vi "Process.vi"(8 "error in (no error)":errorcluster, 10 "Pound in":refnum<class "Pound.lvclass">, 11 "Qbus in":refnum<class "Qbus.lvclass">) -> (0 "error out":errorcluster)   [LabVIEW 2017, in "Controller.lvlib"]
doc: "This process performs device-wide operations, such as restarting all processes during a reboot and monitoring that each process starts up successfully."
uses:
  <vilib>/addons/InsightCM/Devices/Shared/Common/Controller/Controller.lvlib
  <vilib>/addons/Qbus/Qbus.lvclass
  <vilib>/NI/Software Watchdog/Pound/Pound.lvclass
  <vilib>/addons/InsightCM/Devices/Shared/Common/Controller/controls/config.ctl
  <vilib>/addons/BlinkProcess/controls/mode.ctl
  <vilib>/addons/InsightCM/MessageBus/MessageLibrary/Device/controls/DeviceInvalidConfigurationBroadcastBody.ctl
  <vilib>/addons/InsightCM/Devices/Shared/Common/ServerComm/controls/ConnectionStatus.ctl
  <vilib>/addons/InsightCM/Devices/Shared/Cms/CmsAcquisition/controls/StopAcquisitionRequest.ctl
  <vilib>/addons/InsightCM/Devices/Shared/Common/Controller/controls/operations.ctl
  <vilib>/addons/TraceLogger/TraceLogger.lvlib
  <vilib>/NI/Software Watchdog/Watchdog/Watchdog.lvclass
  <vilib>/addons/InsightCM/Devices/Shared/Common/ServerComm/ServerComm.lvlib
  <vilib>/addons/BlinkProcess/BlinkProcess.lvlib
  <vilib>/addons/InsightCM/Utilities/GlobalConfiguration/GlobalConfiguration.lvlib
  <vilib>/addons/InsightCM/Devices/Shared/Cms/CmsAcquisition/CmsAcquisition.lvlib
  <vilib>/addons/InsightCM/Devices/Shared/Cms/CmsBurstMode/BurstMode.lvlib
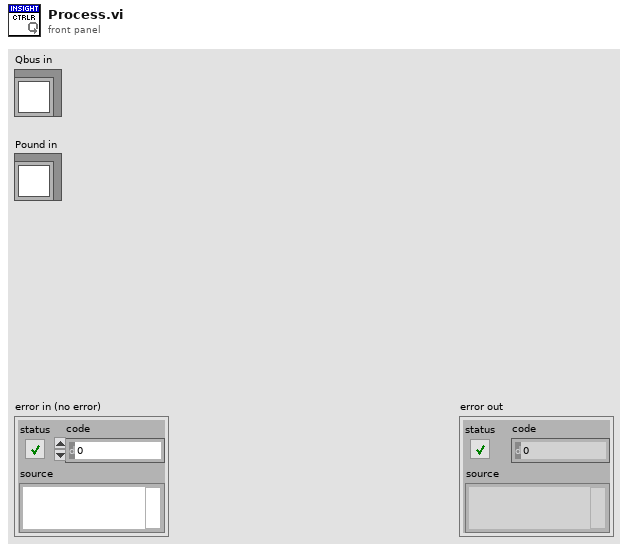
[diagram p1: front panel]
types:
  T1 = typedef "Controller.lvlib/config.ctl" = cluster{"Online":bool, "SafeMode":bool, "InvalidConfig":string, "ShutdownReason":string, "ScheduledShutdown":bool}
  T2 = typedef "BlinkProcess.lvlib/mode.ctl" = enum16{"Normal", "Error", "On", "Off", "Custom"}
  T3 = typedef "DeviceInvalidConfigurationBroadcastBody.ctl" = cluster{"DeviceName":string, "Description":string}
  T4 = typedef "ServerComm.lvlib/ConnectionStatus.ctl" = enum16{"Offline", "NotAuthorized", "Online"}
  T5 = typedef "CmsAcquisition.lvlib/StopAcquisitionRequest.ctl" = cluster{"Reason":string, "State":variant}
  T6 = typedef "Controller.lvlib/operations.ctl" = enum16{"Unknown", "Startup", "Expected Shutdown"}
  T7 = typedef "R2_Device.ctl" = cluster{"Id":string, "Name":string, "DeviceType":string, "HardwareName":string, "IpAddress":string, "HardwareInfo":T8[], "ApplicationType":string, "ApplicationVersion":string, "EquipmentIds":string[], "ConfigurationVersion":string, "State":T9, "Properties":T8[], "DataGroups":T10[], "BurstModeTrigger":T14}
  T8 = typedef "KeyValuePair.ctl" = cluster{"Key":string, "Value":string}
  T9 = typedef "DeviceState.ctl" = cluster{"Disabled":bool}
  T10 = typedef "R2_DataGroup.ctl" = cluster{"Name":string, "OperatingStates":T11[], "Properties":T8[], "EquipmentIds":string[], "AssetNodeId":string}
  T11 = typedef "OperatingState.ctl" = cluster{"Name":string, "Properties":T8[], "Triggers":T12[]}
  T12 = typedef "Trigger.ctl" = cluster{"Type":string, "Expression":string, "Conditions":T13[]}
  T13 = typedef "Condition.ctl" = cluster{"Source":string, "Type":string, "Operator":string, "CompareTo":string, "DwellSeconds":dbl}
  T14 = typedef "BurstModeTrigger.ctl" = cluster{"Trigger":T12, "SampleRate":string, "AcquisitionLength":string}
  T15 = typedef "Message.ctl" = cluster{"Header":T16, "Body":u8[]}
  T16 = typedef "MessageHeader.ctl" = cluster{"MessageName":string, "Timestamp":i64, "CorrelationId":string, "ContentType":string, "RoutingKey":string, "Properties":T8[]}
  T17 = typedef "BurstMode.lvlib/InitiateBurstMode.ctl" = cluster{"Group":string, "Acq Reason":string}
  T18 = typedef "CmsAcquisition.lvlib/StopAcquisitionResponse.ctl" = cluster{"Reason":string, "Acquisition Stopped":bool, "State":variant}
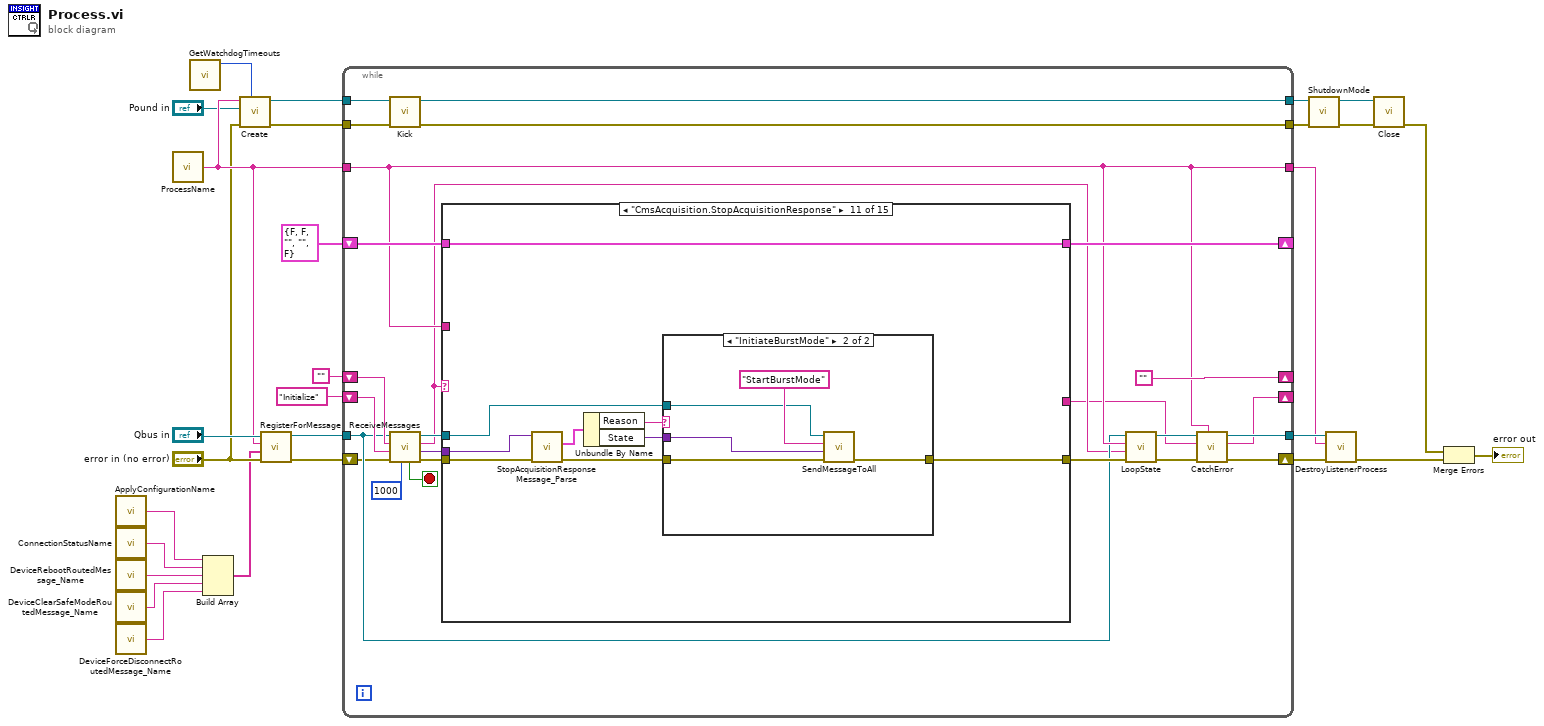
[diagram p0: block diagram]
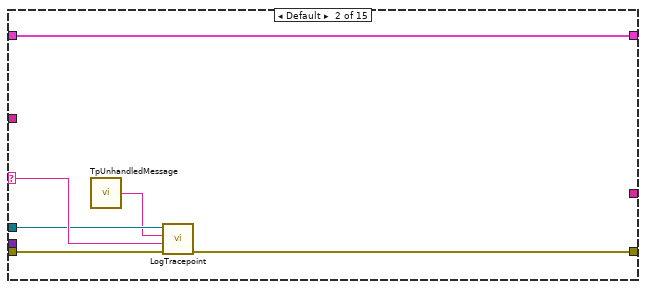
[diagram p3: hidden frame]
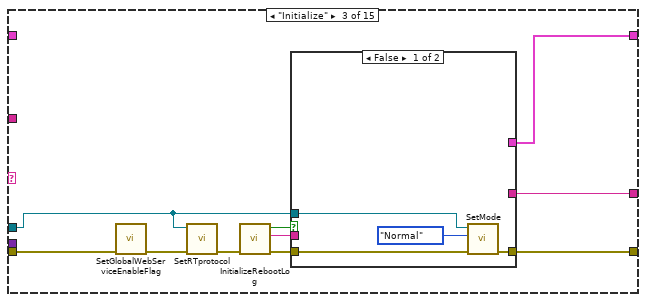
[diagram p4: hidden frame]
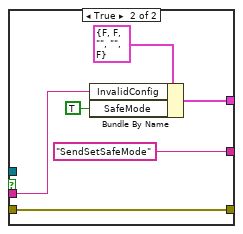
[diagram p5: hidden frame]
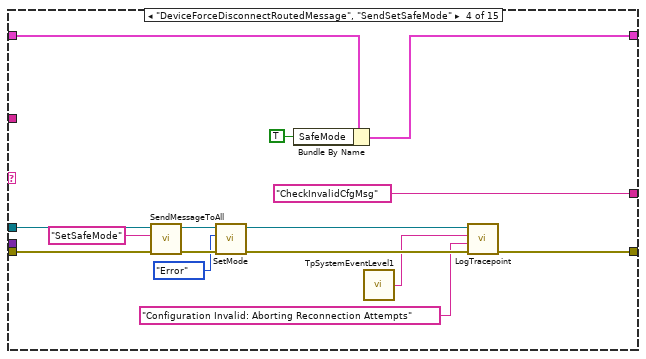
[diagram p6: hidden frame]
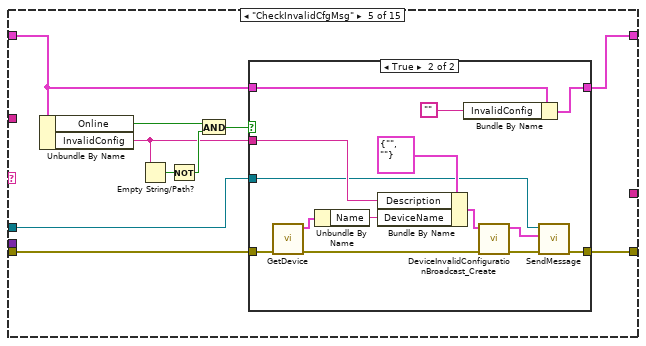
[diagram p7: hidden frame]
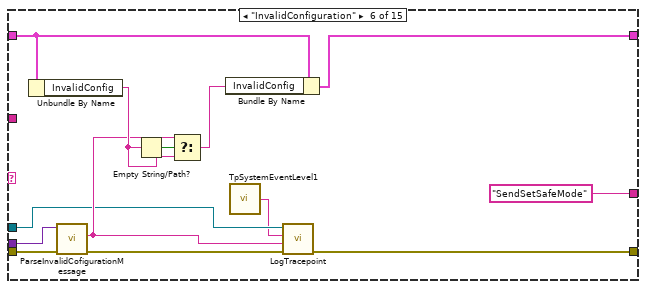
[diagram p9: hidden frame]
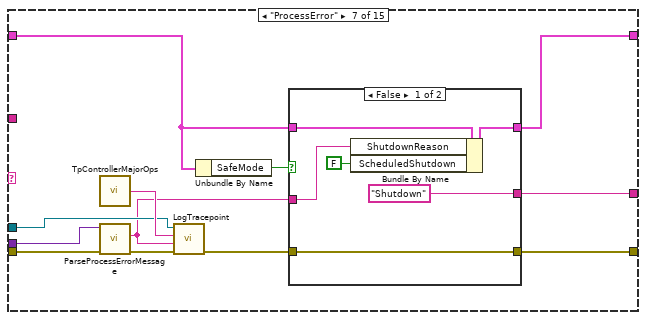
[diagram p10: hidden frame]
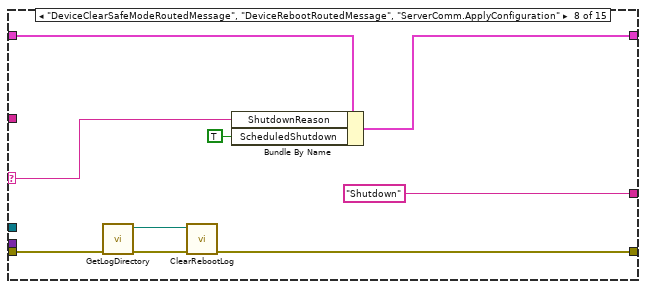
[diagram p12: hidden frame]
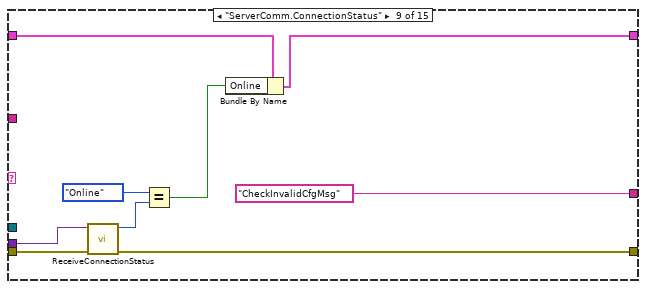
[diagram p13: hidden frame]
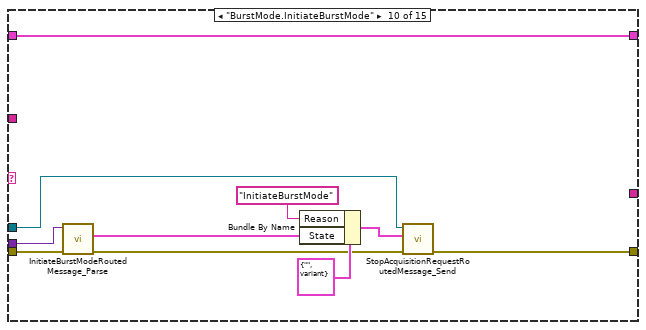
[diagram p14: hidden frame]
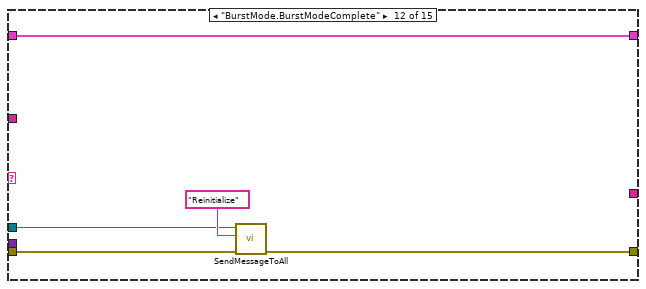
[diagram p16: hidden frame]
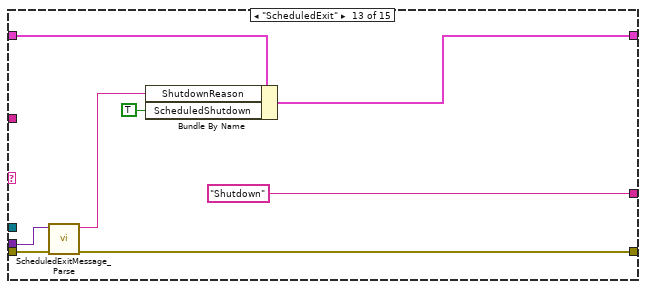
[diagram p17: hidden frame]
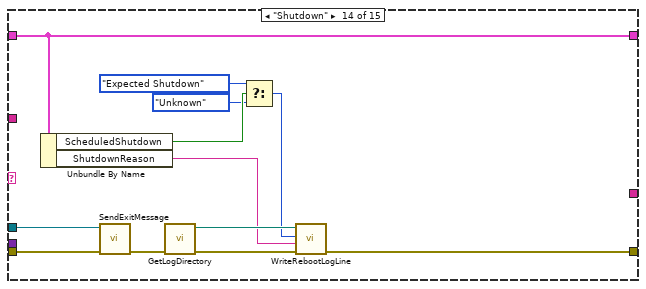
[diagram p18: hidden frame]
diagram:
  n1 = call <vilib>:"ApplyConfigurationName.vi"() -> ("message name"=w6:string)  [unwired: 5 in]
  n2 = call <vilib>:"ConnectionStatusName.vi"() -> ("message name"=w5:string)  [unwired: 5 in]
  n3 = call <vilib>:"DeviceRebootRoutedMessage_Name.vi"() -> ("MessageName"=w4:string)  [unwired: 5 in]
  n4 = call <vilib>:"DeviceClearSafeModeRoutedMessage_Name.vi"() -> ("MessageName"=w3:string)  [unwired: 5 in]
  n5 = call <vilib>:"DeviceForceDisconnectRoutedMessage_Name.vi"() -> ("MessageName"=w2:string)  [unwired: 5 in]
  n6 = call <vilib>:"ProcessName.vi"() -> ("ProcessName"=w19:string)  [unwired: 5 in]
  n7 = call <vilib>:"GetWatchdogTimeouts.vi"() -> ("software timeout"=w1:u32)  [unwired: 10 in, 1 out]
  n8 = Build Array(w6, w5, w4, w3, w2) -> (w7:string[])
  n9 = call <vilib>:"Create.vi"("Execution Timeout (ms)"=w1, "error in (no error)"="error in (no error)", "Pound"="Pound in", "Name"=w19) -> ("error out"=w13:errorcluster, "Watchdog"=w18:refnum<data-value>)  [unwired: 6 in]
  n10 = call <vilib>:"RegisterForMessage.vi"("error in (no error)"="error in (no error)", "message names"=w7, "process name"=w19, "Qbus in"="Qbus in") -> ("error in (no error)"=w27:errorcluster, "Qbus out"=w26:refnum<class "Qbus.lvclass">)  [unwired: 6 in]
  n11 = while {
    shift-right: [""] -> _
    shift-left: "" -> [w52]
    tunnel: w26 -> [w39]
    tunnel: w19 -> [w40]
    tunnel: [w43] -> w24
    tunnel: [w40] -> w23
    shift-right: [w42] -> _
    shift-left: "Initialize" -> [w47]
    shift-right: [w45] -> _
    shift-left: T1 {"Online"=FALSE, "SafeMode"=FALSE, "InvalidConfig"="", "ShutdownReason"="", "ScheduledShutdown"=FALSE} ("config") -> [w46]
    tunnel: w18 -> [w38]
    tunnel: [w37] -> w15
    tunnel: w13 -> [w36]
    tunnel: [w34] -> w12
    shift-right: [w44] -> w25
    shift-left: w27 -> [w35]
    stop <- w53 stop-if-true
    n12 = call <vilib>:"Kick.vi"("error in (no error)"=w36, "Watchdog"=w38) -> ("error out"=w34:errorcluster, "Watchdog"=w37:refnum<data-value>)  [unwired: 8 in]
    n13 = call <vilib>:"ReceiveMessages.vi"("Timeout(100)"=1000, "error in (no error)"=w35, "Priority Action"=w47, "Default Action"=w52, "Qbus in"=w39) -> ("error out"=w51:errorcluster, "MsgValue"=w48:variant, "Action"=w31:string, "Qbus out"=w49:refnum<class "Qbus.lvclass">, "Exit"=w53:bool)  [unwired: 2 in]
    n14 = case shown="\"CmsAcquisition.StopAcquisitionResponse\"" w31 {
      selector: w31 -> [_ w58 _ _ _ _ _ w156 _ _ _ _ _ _ _]
      tunnel: w51 -> [w54 w60 w65 w92 w106 w135 w144 w159 w173 w176 w188 w200 w211 w221 w224]
      tunnel: w49 -> [_ w57 w66 w91 w99 w124 w141 _ _ w182 w190 w201 _ w219 _]
      tunnel: [w54 w59 w69 w85 w105 w126 w146 w157 w169 w178 w191 w199 w204 w220 w224] -> w41
      tunnel: w48 -> [_ _ _ _ _ w134 w143 _ w172 w177 w189 _ w210 _ _]
      tunnel: w46 -> [w55 w61 _ w89 w98 w133 w137 w163 w171 w183 w192 w203 w208 w217 w225]
      tunnel: [w55 w61 w70 w88 w97 w130 w136 w162 w170 w183 w192 w203 w207 w217 w225] -> w45
      tunnel: w40 -> [_ _ _ _ _ _ _ _ _ _ _ _ _ _ _]
      tunnel: [_ _ w62 "CheckInvalidCfgMsg" ("error string") _ "SendSetSafeMode" ("log string") w138 "Shutdown" ("error string") "CheckInvalidCfgMsg" ("error string") _ _ _ "Shutdown" ("error string") _ _] -> w29
      frame "" {
      }
      frame Default {
        n15 = call <vilib>:"TpUnhandledMessage.vi"() -> ("tracepoint name"=w56:string)  [unwired: 5 in]
        n16 = call <vilib>:"LogTracepoint.vi"("error in (no error)"=w60, "log string"=w58, "tracepoint"=w56, "qbus in"=w57) -> ("error out"=w59:errorcluster)  [unwired: 6 in, 1 out]
      }
      frame "Initialize" {
        n17 = call <vilib>:"SetGlobalWebServiceEnableFlag.vi"("error in (no error)"=w65) -> ("error out"=w68:errorcluster)  [unwired: 10 in]
        n18 = call <vilib>:"SetRTprotocol.vi"("error in (no error)"=w68, "Qbus in"=w66) -> ("error out"=w67:errorcluster)  [unwired: 9 in]
        n19 = call <vilib>:"InitializeRebootLog.vi"("error in (no error)"=w67) -> ("error out"=w71:errorcluster, "log string"=w63:string, "reboot count limit met"=w64:bool)  [unwired: 8 in]
        n20 = case shown="False" w64 {
          tunnel: w71 -> [w75 w77]
          tunnel: [w74 w77] -> w69
          tunnel: w66 -> [w73 _]
          tunnel: [_ w81] -> w70
          tunnel: w63 -> [_ w79]
          tunnel: [_ "SendSetSafeMode" ("log string")] -> w62
          frame False {
            n21 = call <vilib>:"SetMode.vi"("error in (no error)"=w75, "mode"=mode."Normal", "Qbus in"=w73) -> ("error out"=w74:errorcluster)  [unwired: 7 in, 1 out]
          }
          frame True {
            n22 = Bundle By Name(cluster=T1 {"Online"=FALSE, "SafeMode"=FALSE, "InvalidConfig"="", "ShutdownReason"="", "ScheduledShutdown"=FALSE} ("config"), "InvalidConfig"=w79, "SafeMode"=TRUE) -> (w81:T1)
          }
        }
      }
      frame "DeviceForceDisconnectRoutedMessage", "SendSetSafeMode" {
        n23 = call <vilib>:"SendMessageToAll.vi"("error in (no error)"=w92, "message name"="SetSafeMode" ("MsgName"), "Qbus in"=w91) -> ("error in (no error)"=w95:errorcluster, "Qbus out"=w94:refnum<class "Qbus.lvclass">)  [unwired: 7 in]
        n24 = call <vilib>:"SetMode.vi"("error in (no error)"=w95, "mode"=mode."Error", "Qbus in"=w94) -> ("error out"=w86:errorcluster, "Qbus out"=w83:refnum<class "Qbus.lvclass">)  [unwired: 7 in]
        n25 = Bundle By Name(cluster=w89, "SafeMode"=TRUE) -> (w88:T1)
        n26 = call <vilib>:"TpSystemEventLevel1.vi"() -> ("tracepoint name"=w84:string)  [unwired: 5 in]
        n27 = call <vilib>:"LogTracepoint.vi"("error in (no error)"=w86, "log string"="Configuration Invalid: Aborting Reconnection Attempts", "tracepoint"=w84, "qbus in"=w83) -> ("error out"=w85:errorcluster)  [unwired: 6 in, 1 out]
      }
      frame "CheckInvalidCfgMsg" {
        n28 = Unbundle By Name(w98) -> ("Online"=w102:bool, "InvalidConfig"=w100:string)
        n29 = Empty String/Path?(string/path=w100) -> (empty?=w104:bool)
        n30 = Not(x=w104) -> (.not. x?=w103:bool)
        n31 = And(x=w102, y=w103) -> (x .and. y?=w101:bool)
        n32 = case shown="True" w101 {
          tunnel: w106 -> [w108 w115]
          tunnel: [w108 w114] -> w105
          tunnel: w100 -> [_ w113]
          tunnel: w99 -> [_ w112]
          tunnel: w98 -> [w107 w111]
          tunnel: [w107 w109] -> w97
          frame False {
          }
          frame True {
            n33 = call <vilib>:"GetDevice.vi"("error in (no error)"=w115) -> ("error out"=w116:errorcluster, "device configuration"=w118:T7)  [unwired: 8 in, 1 out]
            n34 = Unbundle By Name(w118) -> ("Name"=w117:string)
            n35 = Bundle By Name(cluster=T3 {"DeviceName"="", "Description"=""} ("DeviceInvalidConfigurationBroadcast"), "Description"=w113, "DeviceName"=w117) -> (w119:T3)
            n36 = Bundle By Name(cluster=w111, "InvalidConfig"="") -> (w109:T1)
            n37 = call <vilib>:"DeviceInvalidConfigurationBroadcast_Create.vi"("error in (no error)"=w116, "DeviceInvalidConfigurationBroadcast"=w119) -> ("error out"=w121:errorcluster, "Message"=w122:T15)  [unwired: 8 in]
            n38 = call <vilib>:"SendMessage.vi"("error in (no error)"=w121, "message"=w122, "Qbus in"=w112) -> ("error out"=w114:errorcluster)  [unwired: 7 in, 1 out]
          }
        }
      }
      frame "InvalidConfiguration" {
        n39 = Unbundle By Name(w133) -> ("InvalidConfig"=w131:string)
        n40 = call <vilib>:"ParseInvalidCofigurationMessage.vi"("error in (no error)"=w135, "process error message"=w134) -> ("error out"=w127:errorcluster, "description"=w125:string)  [unwired: 8 in]
        n41 = Empty String/Path?(string/path=w131) -> (empty?=w132:bool)
        n42 = Select(t=w125, s=w132, f=w131) -> (s? t:f=w129:string)
        n43 = Bundle By Name(cluster=w133, "InvalidConfig"=w129) -> (w130:T1)
        n44 = call <vilib>:"TpSystemEventLevel1.vi"() -> ("tracepoint name"=w123:string)  [unwired: 5 in]
        n45 = call <vilib>:"LogTracepoint.vi"("error in (no error)"=w127, "log string"=w125, "tracepoint"=w123, "qbus in"=w124) -> ("error out"=w126:errorcluster)  [unwired: 6 in, 1 out]
      }
      frame "ProcessError" {
        n46 = call <vilib>:"TpControllerMajorOps.vi"() -> ("TracepointName"=w147:string)  [unwired: 5 in]
        n47 = call <vilib>:"ParseProcessErrorMessage.vi"("error in (no error)"=w144, "process error message"=w143) -> ("error out"=w142:errorcluster, "error string"=w139:string)  [unwired: 8 in]
        n48 = call <vilib>:"LogTracepoint.vi"("error in (no error)"=w142, "log string"=w139, "tracepoint"=w147, "qbus in"=w141) -> ("error out"=w145:errorcluster)  [unwired: 6 in, 1 out]
        n49 = Unbundle By Name(w137) -> ("SafeMode"=w140:bool)
        n50 = case shown="False" w140 {
          tunnel: [w148 w155] -> w146
          tunnel: w145 -> [w148 w155]
          tunnel: w137 -> [w153 w154]
          tunnel: w139 -> [w152 _]
          tunnel: ["Shutdown" ("error string") _] -> w138
          tunnel: [w149 w154] -> w136
          frame False {
            n51 = Bundle By Name(cluster=w153, "ShutdownReason"=w152, "ScheduledShutdown"=FALSE) -> (w149:T1)
          }
          frame True {
          }
        }
      }
      frame "DeviceClearSafeModeRoutedMessage", "DeviceRebootRoutedMessage", "ServerComm.ApplyConfiguration" {
        n52 = call <vilib>:"GetLogDirectory.vi"("error in (no error)"=w159) -> ("error out"=w158:errorcluster, "log dir"=w160:path)  [unwired: 9 in]
        n53 = call <vilib>:"ClearRebootLog.vi"("error in"=w158, "log path"=w160) -> ("error out"=w157:errorcluster)  [unwired: 9 in]
        n54 = Bundle By Name(cluster=w163, "ShutdownReason"=w156, "ScheduledShutdown"=TRUE) -> (w162:T1)
      }
      frame "ServerComm.ConnectionStatus" {
        n55 = call <vilib>:"ReceiveConnectionStatus.vi"("error in (no error)"=w173, "body"=w172) -> ("error out"=w169:errorcluster, "status"=w168:T4)  [unwired: 6 in, 2 out]
        n56 = Equal?(x=ConnectionStatus."Online" ("status"), y=w168) -> (x = y?=w166:bool)
        n57 = Bundle By Name(cluster=w171, "Online"=w166) -> (w170:T1)
      }
      frame "BurstMode.InitiateBurstMode" {
        n58 = call <vilib>:"InitiateBurstModeRoutedMessage_Parse.vi"("error in (no error)"=w176, "message"=w177) -> ("error out"=w175:errorcluster, "InitiateBurstMode"=w174:T17)  [unwired: 8 in]
        n59 = Bundle By Name(cluster=T5 {"Reason"="", "State"=variant} ("StopAcquisitionRequest"), "Reason"="InitiateBurstMode" ("MsgName"), "State"=w174) -> (w181:T5)
        n60 = call <vilib>:"StopAcquisitionRequestRoutedMessage_Send.vi"("error in (no error)"=w175, "StopAcquisitionRequest"=w181, "Qbus in"=w182) -> ("error out"=w178:errorcluster)  [unwired: 7 in, 1 out]
      }
      frame "CmsAcquisition.StopAcquisitionResponse" {
        n61 = call <vilib>:"StopAcquisitionResponseMessage_Parse.vi"("error in (no error)"=w188, "message"=w189) -> ("error out"=w187:errorcluster, "Stop Acquisition Response"=w186:T18)  [unwired: 8 in]
        n62 = Unbundle By Name(w186) -> ("Reason"=w185:string, "State"=w184:variant)
        n63 = case shown="\"InitiateBurstMode\"" w185 {
          tunnel: [w193 w197] -> w191
          tunnel: w190 -> [_ w196]
          tunnel: w187 -> [w193 w195]
          tunnel: w184 -> [_ w194]
          frame "False", Default {
          }
          frame "InitiateBurstMode" {
            n64 = call <vilib>:"SendMessageToAll.vi"("error in (no error)"=w195, "message value"=w194, "message name"="StartBurstMode" ("MsgName"), "Qbus in"=w196) -> ("error in (no error)"=w197:errorcluster)  [unwired: 6 in, 1 out]
          }
        }
      }
      frame "BurstMode.BurstModeComplete" {
        n65 = call <vilib>:"SendMessageToAll.vi"("error in (no error)"=w200, "message name"="Reinitialize" ("MsgName"), "Qbus in"=w201) -> ("error in (no error)"=w199:errorcluster)  [unwired: 7 in, 1 out]
      }
      frame "ScheduledExit" {
        n66 = call <vilib>:"ScheduledExitMessage_Parse.vi"("error in (no error)"=w211, "scheduled exit message"=w210) -> ("error out"=w204:errorcluster, "scheduled exit reason"=w206:string)  [unwired: 8 in]
        n67 = Bundle By Name(cluster=w208, "ShutdownReason"=w206, "ScheduledShutdown"=TRUE) -> (w207:T1)
      }
      frame "Shutdown" {
        n68 = Unbundle By Name(w217) -> ("ScheduledShutdown"=w216:bool, "ShutdownReason"=w213:string)
        n69 = call <vilib>:"SendExitMessage.vi"("error in (no error)"=w221, "Qbus in"=w219) -> ("error in (no error)"=w223:errorcluster)  [unwired: 8 in, 1 out]
        n70 = call <vilib>:"GetLogDirectory.vi"("error in (no error)"=w223) -> ("error out"=w222:errorcluster, "log dir"=w218:path)  [unwired: 9 in]
        n71 = Select(t=operations."Expected Shutdown" ("operation"), s=w216, f=operations."Unknown" ("operation")) -> (s? t:f=w212:T6)
        n72 = call <vilib>:"WriteRebootLogLine.vi"("error in"=w222, "reboot log text"=w213, "operation"=w212, "log path"=w218) -> ("error out"=w220:errorcluster)  [unwired: 6 in, 1 out]
      }
      frame "Exit" {
      }
    }
    n73 = call <vilib>:"LoopState.vi"("error in (no error)"=w41, "loop action"=w31, "process name"=w40, "Qbus in"=w39) -> ("error out"=w33:errorcluster, "Qbus out"=w32:refnum<class "Qbus.lvclass">)  [unwired: 6 in]
    n74 = call <vilib>:"CatchError.vi"("source"=w40, "error in (no error)"=w33, "next action in"=w29, "Qbus in"=w32) -> ("error out"=w44:errorcluster, "next action out"=w42:string, "Qbus out"=w43:refnum<class "Qbus.lvclass">)  [unwired: 5 in]
  }
  n75 = call <vilib>:"ShutdownMode.vi"("error in (no error)"=w12, "Watchdog"=w15) -> ("error out"=w14:errorcluster, "Watchdog"=w16:refnum<data-value>)  [unwired: 8 in]
  n76 = call <vilib>:"DestroyListenerProcess.vi"("error in (no error)"=w25, "process name"=w23, "Qbus in"=w24) -> ("error in (no error)"=w11:errorcluster)  [unwired: 7 in, 1 out]
  n77 = call <vilib>:"Close.vi"("error in (no error)"=w14, "Watchdog"=w16) -> ("error out"=w10:errorcluster)  [unwired: 9 in]
  n78 = Merge Errors(w10, w11) -> (→"error out":errorcluster)
